vi "LoadScanSettings.vi"(10 "Digitizer Settings In":T1={"Digitizer delay (us) "=0.0, "rf points per line"=2048, "lines per plane"=128, "Samp Rate (Hz)"=100000000.0, "Additional dig delay (us)"=0.0, "Voltage Scale"=0.4, "Pre-Looks"=0, "Offset delay (us)"=0.0, "bits A/D"=8, "Avg Num"=1, "DigTimeOut"=5.0, "Rel Dig Delay"=0.0, "Dig Ch"=0, "LeCroyCluster"={"LeCroy Channels"=[TRUE, FALSE, FALSE, FALSE], "LC read pt offset"=0.0, "Sweep Avg"=FALSE}, "Main Digitizer"=enum."NI Digitizer", "Dig Config"=enum."Single channel", "Digitizer ID Cluster"={"Acqiris/Alazar/SP ID"=[], "NI Instr Handles"=[], "LeCroy VISA"="", "GaGe Handle"={"Handle"=0, "Sample size"=0, "Resolution"=0, "Offset"=0, "Channels"=0, "Boards"=0}, "ATS Ref"="ATS9350", "Acqiris Address"=["PCI::INSTR0"], "ADQRef"=refnum, "adq_cu_ptr"=refnum}, "Trigger Settings"={"Trig Source"=1, "Trig Coupling"=0, "Trig Slope"=0, "Level (mV)"=1500.0}, "Bulk Acq"=FALSE, "Bulk Start Indexes"=[], "Data Ref RF"=refnum, "NI ID/Channel"=[], "Total Dig CH"=5, "Xtra Ann Trig delay (us)"=10.0, "Fix Z Delay?"=FALSE, "One Way Transmission?"=FALSE, "Data Ref Log"=refnum} {"Trigger Settings"."Trig Slope" items=["Positive", "Negative"]; "Trigger Settings"."Level (mV)" format="%.2f"; "Trigger Settings"."Trig Coupling" items=["DC 1 MOhm", "AC 1 MOhm", "DC 50 Ohm", "AC 50 Ohm"]; "Trigger Settings"."Trig Source" items=["Chan 1", "External"]; "Rel Dig Delay" format="%.2f"; "DigTimeOut" format="%.2f"; "Avg Num" min=1; "Offset delay (us)" format="%.2f"; "Additional dig delay (us)" format="%.2f"; "Digitizer delay (us)" format="%.2f"}, 11 "Motion Settings In":T5={"No Motion?"=FALSE, "Motion System"=enum."NI 735x", "Motion Bd ID"=1, "Motion Profile"="SMAC1", "# Axis"=1, "Reverse Z axis?"=TRUE, "SMAC Axis"=0, "scan pair"=enum."y-(x) scan", "RT fps"=6.0, "Steps per mm"=[1000, 1000, 1000, 1000], "Motor Parameters"={"velocity ct/s"=[10000.0, 10000.0, 10000.0, 50000.0], "accel ct/s^2"=[50000.0, 50000.0, 50000.0, 200000.0]}, "One Way Scan"=FALSE, "Reverse One Way Scan"=FALSE, "Global Position (mm)"=[], "Plane"=0, "Distance between\nscan lines (um)"=0.0, "Distance between\nscan planes (um)"=0.0, "number of scan planes"=1, "Total steps in line"=0, "Xtra plane\ndistance  (um)"=100, "Xtra planes "=1, "Add Axis"=FALSE, "overshoot cts"=200, "BKPT Shift"=0, "Scan Start Time (ms)"=0, "ESP VISA"="GPIB::1::INSTR", "3rd Axis"=1, "GL Ref Out"=refnum, "Galil Address"=""} {"3rd Axis" items=["x", "y", "z", "w"]; "Xtra planes" min=1; "Xtra plane\ndistance  (um)" min=0; "Distance between\nscan planes (um)" format="%.2f"; "Distance between\nscan lines (um)" format="%.2f"; "SMAC Axis" items=["None"=0, "Axis 1"=1, "Axis 2"=2, "Axis 3"=3, "Axis 4"=4, "Axis 5"=5, "Axis 6"=6, "Axis 7"=7, "Axis 8"=8, "Vector Space 1"=17, "Vector Space 2"=18, "Vector Space 3"=19, "Vector Space 4"=20]; "Motion Bd ID" min=1 max=32 step=1}) -> (0 "Canceled":bool, 1 "Type of scan out":T13=enum."M scan", 2 "Digitizer Settings out":T1={"Digitizer delay (us) "=0.0, "rf points per line"=2048, "lines per plane"=128, "Samp Rate (Hz)"=100000000.0, "Additional dig delay (us)"=0.0, "Voltage Scale"=0.4, "Pre-Looks"=0, "Offset delay (us)"=0.0, "bits A/D"=8, "Avg Num"=1, "DigTimeOut"=5.0, "Rel Dig Delay"=0.0, "Dig Ch"=0, "LeCroyCluster"={"LeCroy Channels"=[TRUE, FALSE, FALSE, FALSE], "LC read pt offset"=0.0, "Sweep Avg"=FALSE}, "Main Digitizer"=enum."NI Digitizer", "Dig Config"=enum."Single channel", "Digitizer ID Cluster"={"Acqiris/Alazar/SP ID"=[], "NI Instr Handles"=[], "LeCroy VISA"="", "GaGe Handle"={"Handle"=0, "Sample size"=0, "Resolution"=0, "Offset"=0, "Channels"=0, "Boards"=0}, "ATS Ref"="ATS9350", "Acqiris Address"=["PCI::INSTR0"], "ADQRef"=refnum, "adq_cu_ptr"=refnum}, "Trigger Settings"={"Trig Source"=1, "Trig Coupling"=0, "Trig Slope"=0, "Level (mV)"=1500.0}, "Bulk Acq"=FALSE, "Bulk Start Indexes"=[], "Data Ref RF"=refnum, "NI ID/Channel"=[], "Total Dig CH"=5, "Xtra Ann Trig delay (us)"=10.0, "Fix Z Delay?"=FALSE, "One Way Transmission?"=FALSE, "Data Ref Log"=refnum} {"Trigger Settings"."Trig Slope" items=["Positive", "Negative"]; "Trigger Settings"."Level (mV)" format="%.2f"; "Trigger Settings"."Trig Coupling" items=["DC 1 MOhm", "AC 1 MOhm", "DC 50 Ohm", "AC 50 Ohm"]; "Trigger Settings"."Trig Source" items=["Chan 1", "External"]; "Rel Dig Delay" format="%.2f"; "DigTimeOut" format="%.2f"; "Avg Num" min=1; "Offset delay (us)" format="%.2f"; "Additional dig delay (us)" format="%.2f"; "Digitizer delay (us)" format="%.2f"}, 3 "Motion Settings out":T5={"No Motion?"=FALSE, "Motion System"=enum."NI 735x", "Motion Bd ID"=1, "Motion Profile"="SMAC1", "# Axis"=1, "Reverse Z axis?"=TRUE, "SMAC Axis"=0, "scan pair"=enum."y-(x) scan", "RT fps"=6.0, "Steps per mm"=[1000, 1000, 1000, 1000], "Motor Parameters"={"velocity ct/s"=[10000.0, 10000.0, 10000.0, 50000.0], "accel ct/s^2"=[50000.0, 50000.0, 50000.0, 200000.0]}, "One Way Scan"=FALSE, "Reverse One Way Scan"=FALSE, "Global Position (mm)"=[], "Plane"=0, "Distance between\nscan lines (um)"=0.0, "Distance between\nscan planes (um)"=0.0, "number of scan planes"=1, "Total steps in line"=0, "Xtra plane\ndistance  (um)"=100, "Xtra planes "=1, "Add Axis"=FALSE, "overshoot cts"=200, "BKPT Shift"=0, "Scan Start Time (ms)"=0, "ESP VISA"="GPIB::1::INSTR", "3rd Axis"=1, "GL Ref Out"=refnum, "Galil Address"=""} {"3rd Axis" items=["x", "y", "z", "w"]; "Xtra planes" min=1; "Xtra plane\ndistance  (um)" min=0; "Distance between\nscan planes (um)" format="%.2f"; "Distance between\nscan lines (um)" format="%.2f"; "SMAC Axis" items=["None"=0, "Axis 1"=1, "Axis 2"=2, "Axis 3"=3, "Axis 4"=4, "Axis 5"=5, "Axis 6"=6, "Axis 7"=7, "Axis 8"=8, "Vector Space 1"=17, "Vector Space 2"=18, "Vector Space 3"=19, "Vector Space 4"=20]; "Motion Bd ID" min=1 max=32 step=1}, 4 "Panametrics Settings Out":T11={"ENERGY (uJ)"=0, "DAMPING (Ohm)"=0, "HP FILT (KHz) "=0, "LP FILT (MHz)"=0, "MODE"=0, "PRF (KHz)"=1, "GAIN (db)"=0, "COARSE ATTENUATION"=0, "FINE ATTENUATION"=0} {"FINE ATTENUATION" items=["00.0", "00.5", "01.0", "01.5", "02.0", "02.5", "03.0", "03.5", "04.0", "04.5", "05.0", "05.5", "06.0", "06.5", "07.0", "07.5", "08.0", "08.5", "09.0", "09.5", "10.0", "10.5", "11.0", "11.5", "12.0", "12.5", "13.0", "13.5", "14.0", "14.5", "15.0", "15.5"]; "COARSE ATTENUATION" items=["00.0", "10.0", "20.0", "30.0", "40.0", "50.0"]; "GAIN (db)" items=["26.0", "40.0", "54.0"]; "PRF (KHz)" items=["XREMT", "EXBNC", "0.200", "0.500", "1.000", "2.000", "5.000", "10.00", "20.00"]; "MODE" items=["P/ E", "THRU", "RPP", "EXT_PLSR"]; "LP FILT (MHz)" items=["20", "50", "100", "200"]; "HP FILT (KHz)" items=["1", "1000", "3000", "10000"]; "DAMPING (Ohm)" items=["7", "10", "16", "20", "26", "30", "40", "50"]; "ENERGY (uJ)" items=["1", "2", "4", "8", "16", "32"]}, 5 "Daxsonics Settings Out":T10={"Freq (MHz) "=20, "Voltage (V)"=0, "Gain (dB)"=22} {"Freq (MHz)" items=["50"=50, "45"=45, "40"=40, "35"=35, "30"=30, "25"=25, "20"=20, "18"=18, "17"=17, "16"=16, "15"=15, "14"=14, "12"=12, "10"=10, "8"=8, "6"=6, "5"=5, "4"=4]; "Voltage (V)" items=["190"=190, "180"=180, "170"=170, "160"=160, "150"=150, "140"=140, "130"=130, "120"=120, "110"=110, "100"=100, "95"=95, "90"=90, "85"=85, "80"=80, "75"=75, "70"=70, "65"=65, "60"=60, "55"=55, "50"=50, "45"=45, "40"=40, "35"=35, "30"=30, "25"=25, "20"=20, "15"=15, "10"=10, "5"=5, "0"=0]; "Gain (dB)" items=["67"=67, "64"=64, "61"=61, "58"=58, "55"=55, "52"=52, "49"=49, "46"=46, "43"=43, "40"=40, "37"=37, "34"=34, "31"=31, "28"=28, "25"=25, "22"=22]}, 6 "Case Name Modifier Out":string, 8 "Pulser Out":T9)   [LabVIEW 2022 SP3]
uses:
  Controls/ScanType2.ctl
  Motion Controllers/-MotionRoutines/ScanAxis.ctl
  Motion Controllers/NI_controller/-NI_MotionRoutines/MotionParameters.ctl
  Motion Controllers/NI_controller/-NI_MotionRoutines/MotionSys.ctl
  Motion Controllers/-MotionRoutines/3rdAxis.ctl
  Digitizers/-DigitizerRoutines/DigitizerSettings.ctl
  Digitizers/-DigitizerRoutines/Digitizer.ctl
  Digitizers/-DigitizerRoutines/DigConfig.ctl
  Digitizers/-DigitizerRoutines/DigitizerID.ctl
  C:/Windows/System32/ADQAPI_dotNet_helper.dll
  Controls/CompleteScanSettings.ctl
  Pulsers/Panametrics/Pana5900.ctl
  Pulsers/Daxsonics/-DaxSubroutines/Dax_Control_Cluster.ctl
  Pulsers/pulser.ctl
  Motion Controllers/-MotionRoutines/MotionGlobals.vi
  <vilib>/Utility/xml.llb/Read From XML File(string).vi
panel:
  in  "Cancel":bool
  in  "Daxsonics Settings":T10={"Freq (MHz) "=20, "Voltage (V)"=0, "Gain (dB)"=22} {"Freq (MHz)" items=["50"=50, "45"=45, "40"=40, "35"=35, "30"=30, "25"=25, "20"=20, "18"=18, "17"=17, "16"=16, "15"=15, "14"=14, "12"=12, "10"=10, "8"=8, "6"=6, "5"=5, "4"=4]; "Voltage (V)" items=["190"=190, "180"=180, "170"=170, "160"=160, "150"=150, "140"=140, "130"=130, "120"=120, "110"=110, "100"=100, "95"=95, "90"=90, "85"=85, "80"=80, "75"=75, "70"=70, "65"=65, "60"=60, "55"=55, "50"=50, "45"=45, "40"=40, "35"=35, "30"=30, "25"=25, "20"=20, "15"=15, "10"=10, "5"=5, "0"=0]; "Gain (dB)" items=["67"=67, "64"=64, "61"=61, "58"=58, "55"=55, "52"=52, "49"=49, "46"=46, "43"=43, "40"=40, "37"=37, "34"=34, "31"=31, "28"=28, "25"=25, "22"=22]}
  in  "Panametrics Settings":T11={"ENERGY (uJ)"=0, "DAMPING (Ohm)"=0, "HP FILT (KHz) "=0, "LP FILT (MHz)"=0, "MODE"=0, "PRF (KHz)"=1, "GAIN (db)"=0, "COARSE ATTENUATION"=0, "FINE ATTENUATION"=0} {"FINE ATTENUATION" items=["00.0", "00.5", "01.0", "01.5", "02.0", "02.5", "03.0", "03.5", "04.0", "04.5", "05.0", "05.5", "06.0", "06.5", "07.0", "07.5", "08.0", "08.5", "09.0", "09.5", "10.0", "10.5", "11.0", "11.5", "12.0", "12.5", "13.0", "13.5", "14.0", "14.5", "15.0", "15.5"]; "COARSE ATTENUATION" items=["00.0", "10.0", "20.0", "30.0", "40.0", "50.0"]; "GAIN (db)" items=["26.0", "40.0", "54.0"]; "PRF (KHz)" items=["XREMT", "EXBNC", "0.200", "0.500", "1.000", "2.000", "5.000", "10.00", "20.00"]; "MODE" items=["P/ E", "THRU", "RPP", "EXT_PLSR"]; "LP FILT (MHz)" items=["20", "50", "100", "200"]; "HP FILT (KHz)" items=["1", "1000", "3000", "10000"]; "DAMPING (Ohm)" items=["7", "10", "16", "20", "26", "30", "40", "50"]; "ENERGY (uJ)" items=["1", "2", "4", "8", "16", "32"]}
  in  "Pulser":T9
  in  "ScanSettings":T12={"Type of scan"=enum."M scan", "Motion Settings In"={"No Motion?"=FALSE, "Motion System"=enum."NI 735x", "Motion Bd ID"=1, "Motion Profile"="SMAC1", "# Axis"=1, "Reverse Z axis?"=TRUE, "SMAC Axis"=0, "scan pair"=enum."y-(x) scan", "RT fps"=6.0, "Steps per mm"=[1000, 1000, 1000, 1000], "Motor Parameters"={"velocity ct/s"=[10000.0, 10000.0, 10000.0, 50000.0], "accel ct/s^2"=[50000.0, 50000.0, 50000.0, 200000.0]}, "One Way Scan"=FALSE, "Reverse One Way Scan"=FALSE, "Global Position (mm)"=[], "Plane"=0, "Distance between\nscan lines (um)"=0.0, "Distance between\nscan planes (um)"=0.0, "number of scan planes"=1, "Total steps in line"=0, "Xtra plane\ndistance  (um)"=100, "Xtra planes "=1, "Add Axis"=FALSE, "overshoot cts"=200, "BKPT Shift"=0, "Scan Start Time (ms)"=0, "ESP VISA"="GPIB::1::INSTR", "3rd Axis"=1, "GL Ref Out"=refnum, "Galil Address"=""}, "Digitizer Settings"={"Digitizer delay (us) "=0.0, "rf points per line"=2048, "lines per plane"=128, "Samp Rate (Hz)"=100000000.0, "Additional dig delay (us)"=0.0, "Voltage Scale"=0.4, "Pre-Looks"=0, "Offset delay (us)"=0.0, "bits A/D"=8, "Avg Num"=1, "DigTimeOut"=5.0, "Rel Dig Delay"=0.0, "Dig Ch"=0, "LeCroyCluster"={"LeCroy Channels"=[TRUE, FALSE, FALSE, FALSE], "LC read pt offset"=0.0, "Sweep Avg"=FALSE}, "Main Digitizer"=enum."NI Digitizer", "Dig Config"=enum."Single channel", "Digitizer ID Cluster"={"Acqiris/Alazar/SP ID"=[], "NI Instr Handles"=[], "LeCroy VISA"="", "GaGe Handle"={"Handle"=0, "Sample size"=0, "Resolution"=0, "Offset"=0, "Channels"=0, "Boards"=0}, "ATS Ref"="ATS9350", "Acqiris Address"=["PCI::INSTR0"], "ADQRef"=refnum, "adq_cu_ptr"=refnum}, "Trigger Settings"={"Trig Source"=1, "Trig Coupling"=0, "Trig Slope"=0, "Level (mV)"=1500.0}, "Bulk Acq"=FALSE, "Bulk Start Indexes"=[], "Data Ref RF"=refnum, "NI ID/Channel"=[], "Total Dig CH"=1, "Xtra Ann Trig delay (us)"=10.0, "Fix Z Delay?"=FALSE, "One Way Transmission?"=FALSE, "Data Ref Log"=refnum}, "Case Name Modifier"="Case", "Panametrics Settings"={"ENERGY (uJ)"=0, "DAMPING (Ohm)"=0, "HP FILT (KHz) "=0, "LP FILT (MHz)"=0, "MODE"=0, "PRF (KHz)"=1, "GAIN (db)"=0, "COARSE ATTENUATION"=0, "FINE ATTENUATION"=0}, "Daxsonics Settings"={"Freq (MHz) "=20, "Voltage (V)"=0, "Gain (dB)"=22}, "Pulser"=enum."Pan 5900"} {"Daxsonics Settings"."Freq (MHz)" items=["50"=50, "45"=45, "40"=40, "35"=35, "30"=30, "25"=25, "20"=20, "18"=18, "17"=17, "16"=16, "15"=15, "14"=14, "12"=12, "10"=10, "8"=8, "6"=6, "5"=5, "4"=4]; "Daxsonics Settings"."Voltage (V)" items=["190"=190, "180"=180, "170"=170, "160"=160, "150"=150, "140"=140, "130"=130, "120"=120, "110"=110, "100"=100, "95"=95, "90"=90, "85"=85, "80"=80, "75"=75, "70"=70, "65"=65, "60"=60, "55"=55, "50"=50, "45"=45, "40"=40, "35"=35, "30"=30, "25"=25, "20"=20, "15"=15, "10"=10, "5"=5, "0"=0]; "Daxsonics Settings"."Gain (dB)" items=["67"=67, "64"=64, "61"=61, "58"=58, "55"=55, "52"=52, "49"=49, "46"=46, "43"=43, "40"=40, "37"=37, "34"=34, "31"=31, "28"=28, "25"=25, "22"=22]; "Panametrics Settings"."FINE ATTENUATION" items=["00.0", "00.5", "01.0", "01.5", "02.0", "02.5", "03.0", "03.5", "04.0", "04.5", "05.0", "05.5", "06.0", "06.5", "07.0", "07.5", "08.0", "08.5", "09.0", "09.5", "10.0", "10.5", "11.0", "11.5", "12.0", "12.5", "13.0", "13.5", "14.0", "14.5", "15.0", "15.5"]; "Panametrics Settings"."COARSE ATTENUATION" items=["00.0", "10.0", "20.0", "30.0", "40.0", "50.0"]; "Panametrics Settings"."GAIN (db)" items=["26.0", "40.0", "54.0"]; "Panametrics Settings"."PRF (KHz)" items=["XREMT", "EXBNC", "0.200", "0.500", "1.000", "2.000", "5.000", "10.00", "20.00"]; "Panametrics Settings"."MODE" items=["P/ E", "THRU", "RPP", "EXT_PLSR"]; "Panametrics Settings"."LP FILT (MHz)" items=["20", "50", "100", "200"]; "Panametrics Settings"."HP FILT (KHz)" items=["1", "1000", "3000", "10000"]; "Panametrics Settings"."DAMPING (Ohm)" items=["7", "10", "16", "20", "26", "30", "40", "50"]; "Panametrics Settings"."ENERGY (uJ)" items=["1", "2", "4", "8", "16", "32"]; "Digitizer Settings"."Trigger Settings"."Trig Slope" items=["Positive", "Negative"]; "Digitizer Settings"."Trigger Settings"."Level (mV)" format="%.2f"; "Digitizer Settings"."Trigger Settings"."Trig Coupling" items=["DC 1 MOhm", "AC 1 MOhm", "DC 50 Ohm", "AC 50 Ohm"]; "Digitizer Settings"."Trigger Settings"."Trig Source" items=["Chan 1", "External"]; "Digitizer Settings"."Rel Dig Delay" format="%.2f"; "Digitizer Settings"."DigTimeOut" format="%.2f"; "Digitizer Settings"."Avg Num" min=1; "Digitizer Settings"."Offset delay (us)" format="%.2f"; "Digitizer Settings"."Additional dig delay (us)" format="%.2f"; "Digitizer Settings"."Digitizer delay (us)" format="%.2f"; "Motion Settings In"."3rd Axis" items=["x", "y", "z", "w"]; "Motion Settings In"."Xtra planes" min=1; "Motion Settings In"."Xtra plane\ndistance  (um)" min=0; "Motion Settings In"."Distance between\nscan planes (um)" format="%.2f"; "Motion Settings In"."Distance between\nscan lines (um)" format="%.2f"; "Motion Settings In"."SMAC Axis" items=["None"=0, "Axis 1"=1, "Axis 2"=2, "Axis 3"=3, "Axis 4"=4, "Axis 5"=5, "Axis 6"=6, "Axis 7"=7, "Axis 8"=8, "Vector Space 1"=17, "Vector Space 2"=18, "Vector Space 3"=19, "Vector Space 4"=20]; "Motion Settings In"."Motion Bd ID" min=1 max=32 step=1}
  out "Size of one \nRF line (mm)":dbl=128.0 format="%.2f"
  out "Size of all \nplanes (mm)":dbl=128.0 format="%.2f"
  out "Size of one \nplane (mm)":dbl=128.0 format="%.2f"
  in  "Fix Z Delay?":bool
  in  "Voltage Scale":dbl
  in  "Additional dig delay (us)":dbl
  in  "Digitizer delay (us)":dbl
  in  "Samp Rate (MHz)":dbl
  in  "lines per plane":i32
  in  "rf points per line":i32
  in  "number of scan planes":i32
  in  "Distance between\nscan planes (um)":sgl
  in  "Distance between\nscan lines (um)":sgl
  in  "Reverse One Way Scan":bool
  in  "One Way Scan":bool
  in  "scan pair":T7=enum."x-(y) scan"
  in  "save":bool
  in  "Type of scan":T13=enum."M scan"
  in  "Case Name Modifier":string="Case"
  # "Confirm Relevant Settings"
  # "1-D and 2-D B scan settings"
  # "1-D and 2-D B scan settings"
  # "1-D and 2-D B scan settings"
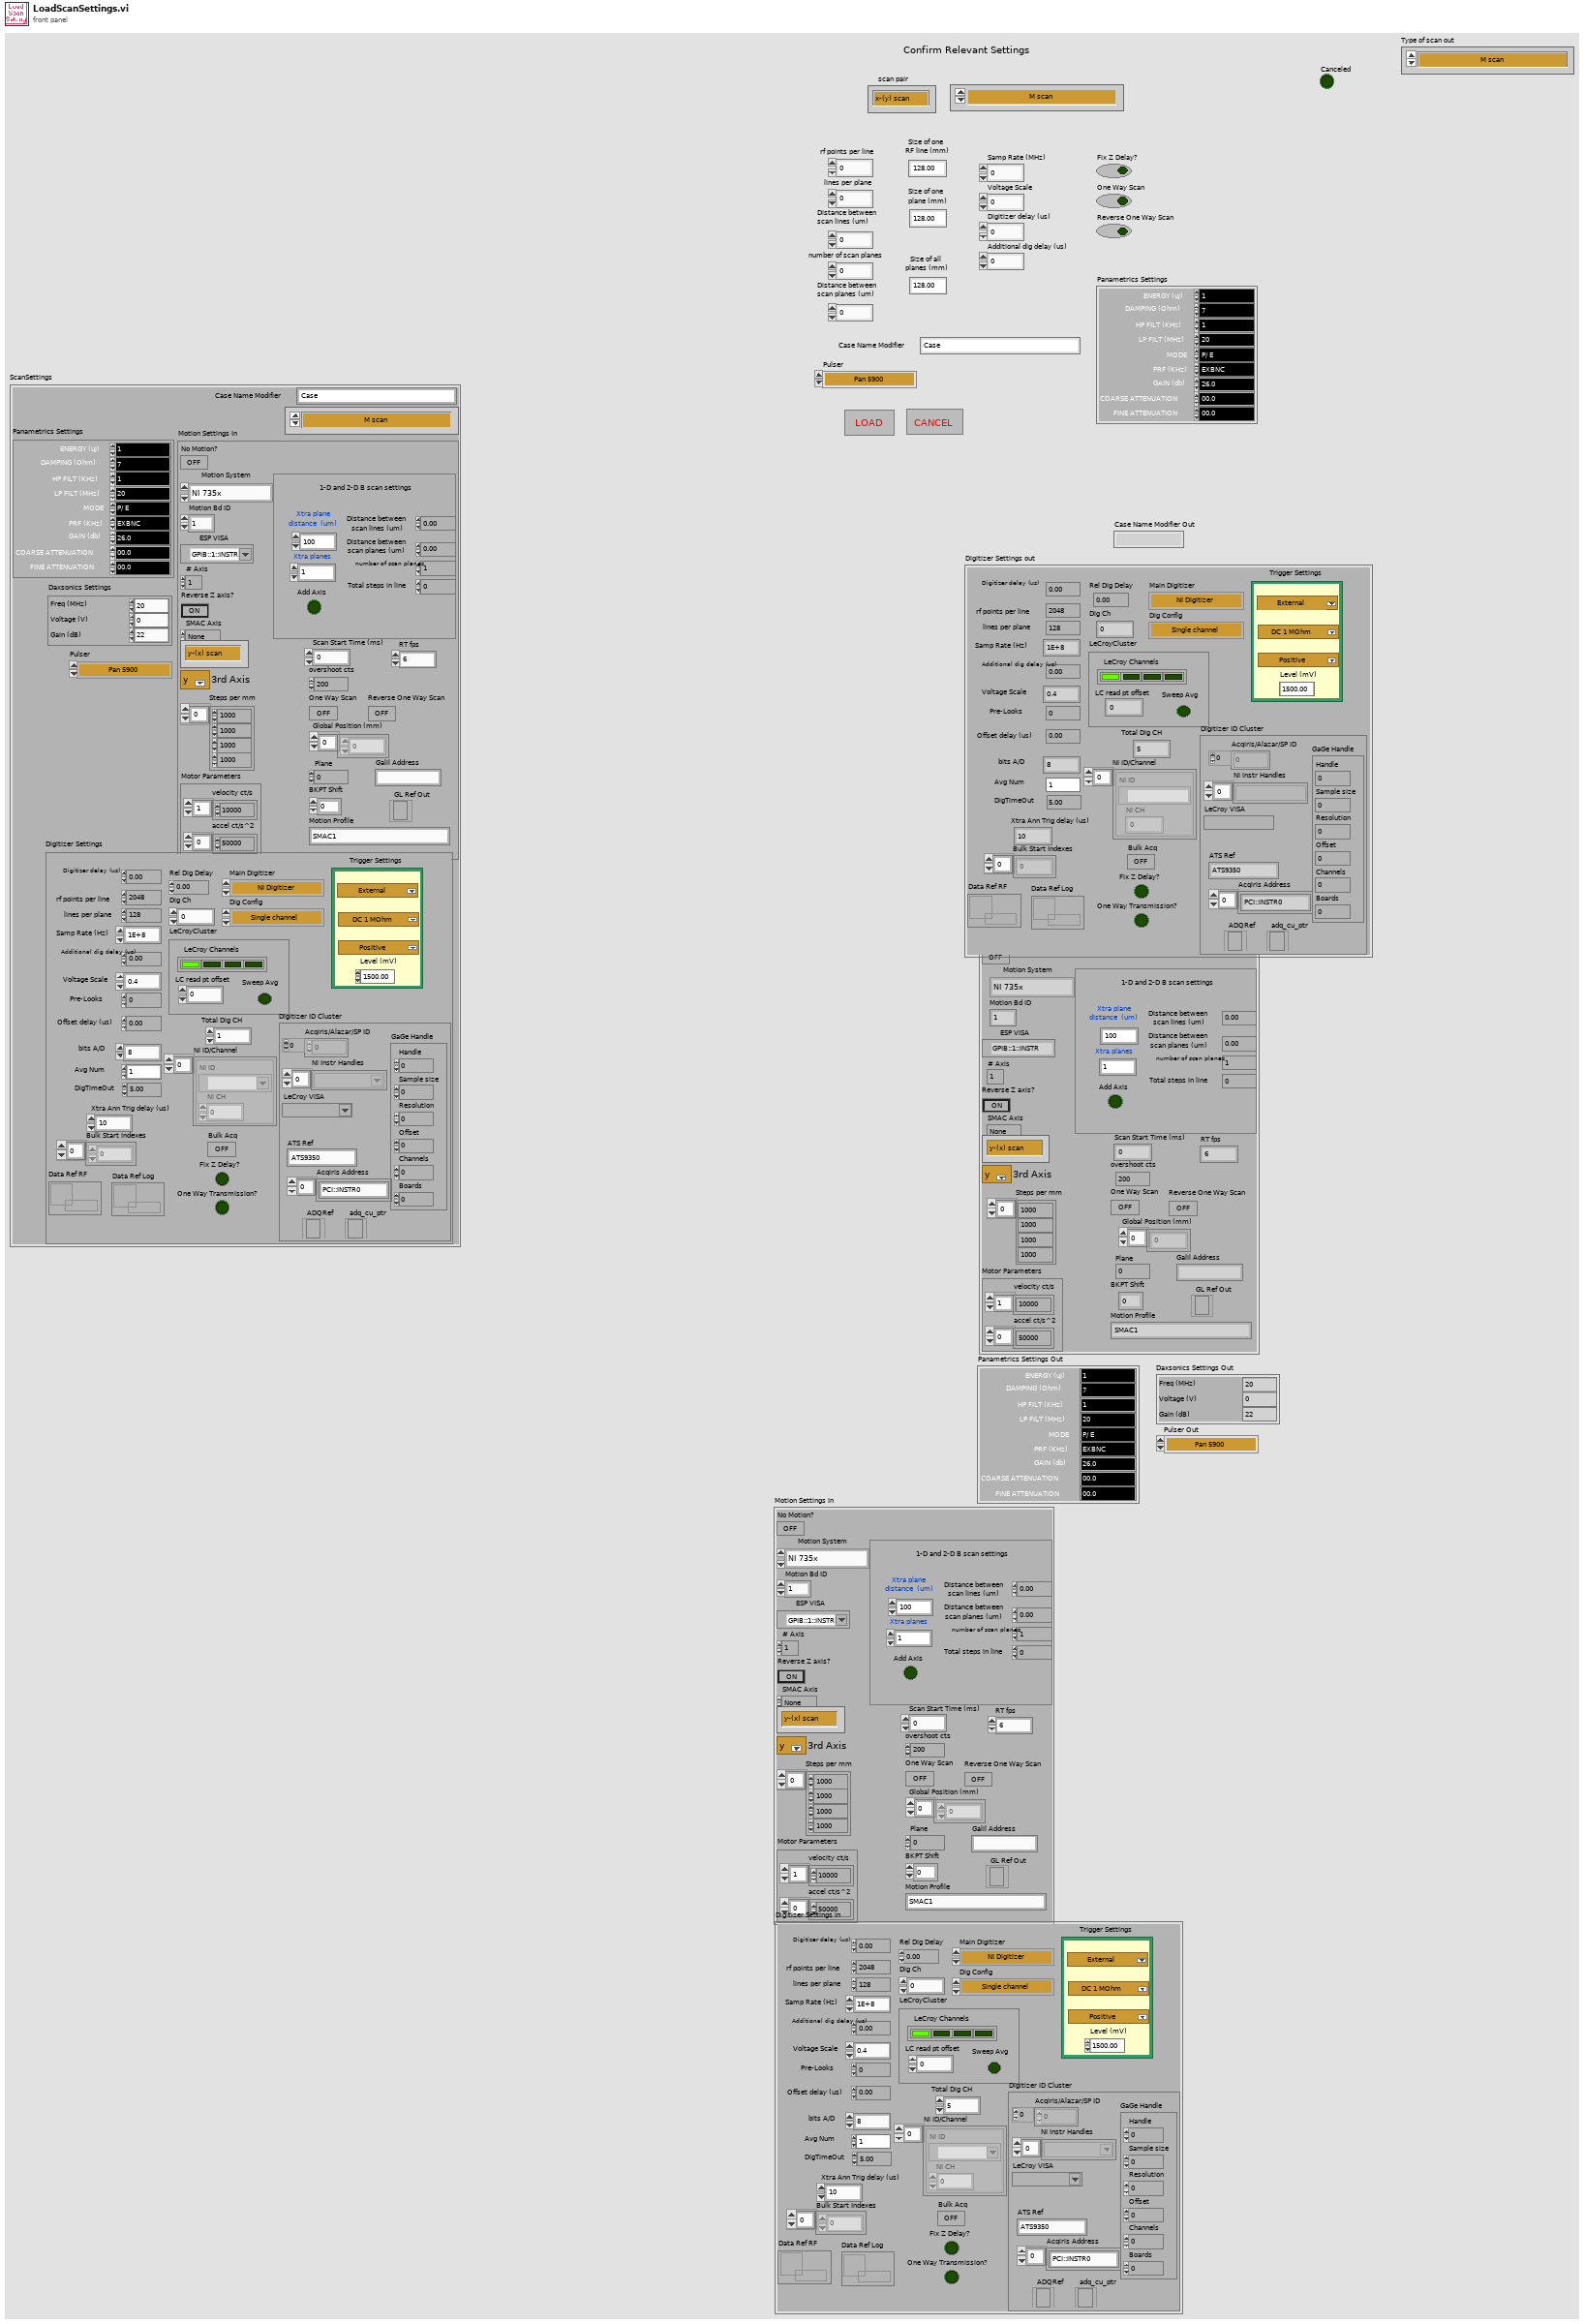
[diagram p1: front panel]
types:
  T1 = typedef "DigitizerSettings.ctl" = cluster{"Digitizer delay (us) ":dbl, "rf points per line":i32, "lines per plane":i32, "Samp Rate (Hz)":dbl, "Additional dig delay (us)":dbl, "Voltage Scale":dbl, "Pre-Looks":i32, "Offset delay (us)":dbl, "bits A/D":i8, "Avg Num":i32, "DigTimeOut":sgl, "Rel Dig Delay":sgl, "Dig Ch":i32, "LeCroyCluster":cluster{"LeCroy Channels":bool[], "LC read pt offset":dbl, "Sweep Avg":bool}, "Main Digitizer":T2, "Dig Config":T3, "Digitizer ID Cluster":T4, "Trigger Settings":cluster{"Trig Source":u16, "Trig Coupling":u16, "Trig Slope":u16, "Level (mV)":dbl}, "Bulk Acq":bool, "Bulk Start Indexes":i32[], "Data Ref RF":refnum<data-value>, "NI ID/Channel":cluster{"NI ID":refnum<k15>, "NI CH":i32}[], "Total Dig CH":i32, "Xtra Ann Trig delay (us)":dbl, "Fix Z Delay?":bool, "One Way Transmission?":bool, "Data Ref Log":refnum<data-value>}
  T2 = typedef "Digitizer.ctl" = enum16{"Acqiris Digitizer", "NI Digitizer", "LeCroy", "GaGe", "AlazarTech", "No Digitizer", "Teledyne"}
  T3 = typedef "DigConfig.ctl" = enum16{"Single channel", "2 Chans w/ 2 Acqiris", "2 Chans w/ 1 Acqiris", "5-CH Pulser New", "5-CH pulser w/ ann array", "5-pass style ann array", "Empty"}
  T4 = typedef "DigitizerID.ctl" = cluster{"Acqiris/Alazar/SP ID":u32[], "NI Instr Handles":refnum<k15>[], "LeCroy VISA":refnum<visa-resource-name>, "GaGe Handle":cluster{"Handle":u32, "Sample size":u32, "Resolution":i32, "Offset":i32, "Channels":u32, "Boards":u32}, "ATS Ref":string, "Acqiris Address":string[], "ADQRef":refnum<k24>, "adq_cu_ptr":refnum<k24>}
  T5 = typedef "MotionParameters.ctl" = cluster{"No Motion?":bool, "Motion System":T6, "Motion Bd ID":u8, "Motion Profile":string, "# Axis":i8, "Reverse Z axis?":bool, "SMAC Axis":u16, "scan pair":T7, "RT fps":sgl, "Steps per mm":i32[], "Motor Parameters":cluster{"velocity ct/s":dbl[], "accel ct/s^2":dbl[]}, "One Way Scan":bool, "Reverse One Way Scan":bool, "Global Position (mm)":dbl[], "Plane":i32, "Distance between\nscan lines (um)":sgl, "Distance between\nscan planes (um)":sgl, "number of scan planes":i32, "Total steps in line":i32, "Xtra plane\ndistance  (um)":i32, "Xtra planes ":i32, "Add Axis":bool, "overshoot cts":i32, "BKPT Shift":i32, "Scan Start Time (ms)":u32, "ESP VISA":refnum<visa-resource-name>, "3rd Axis":T8, "GL Ref Out":refnum<k7>, "Galil Address":string}
  T6 = typedef "MotionSys.ctl" = enum16{"MM3000", "NI 735x", "Newport ESP", "No Motion Card", "Galil"}
  T7 = typedef "ScanAxis.ctl" = enum16{"y-(x) scan", "x-(y) scan", "z-(x) scan", "z-(y) scan", "y-(z) scan", "x-(z) scan", "w-(x) scan", "w-(y) scan", "w-(z) scan", "x-(w) scan", "y-(w) scan", "z-(w) scan"}
  T8 = typedef "3rdAxis.ctl" = u16
  T9 = typedef "pulser.ctl" = enum16{"Pan 5900", "Daxsonics", "Agilent 33xxx", "UTEX", "JSR", "WMC Mono-Cycle", "No Pulser", "NYU AVTECH", "Tabor W1281A", "Pan 5800", "Unlisted", "Tabor WX2182B"}
  T10 = typedef "Dax_Control_Cluster.ctl" = cluster{"Freq (MHz) ":u16, "Voltage (V)":u16, "Gain (dB)":u16}
  T11 = typedef "Pana5900.ctl" = cluster{"ENERGY (uJ)":u16, "DAMPING (Ohm)":u16, "HP FILT (KHz) ":u16, "LP FILT (MHz)":u16, "MODE":u16, "PRF (KHz)":u16, "GAIN (db)":u16, "COARSE ATTENUATION":u16, "FINE ATTENUATION":u16}
  T12 = typedef "CompleteScanSettings.ctl" = cluster{"Type of scan":T13, "Motion Settings In":T5, "Digitizer Settings":T1, "Case Name Modifier":string, "Panametrics Settings":T11, "Daxsonics Settings":T10, "Pulser":T9}
  T13 = typedef "ScanType2.ctl" = enum16{"Therapy With Scan", "M scan", "M Scan With Therapy Burst", "1-D B Scan", "1-D B Scan With Therapy Burst", "2-D B Scan", "2-D B Scan With Therapy Burst", "Rotational Scan", "1-D B-Scan PRF", "2-D B-Scan PRF", "Real-Time Scan", "Contrast Agents", "1-D w/ Real-Time Set Up", "Dual Transducer", "Acoustic Microscopy", "Hydrophone Scanning"}
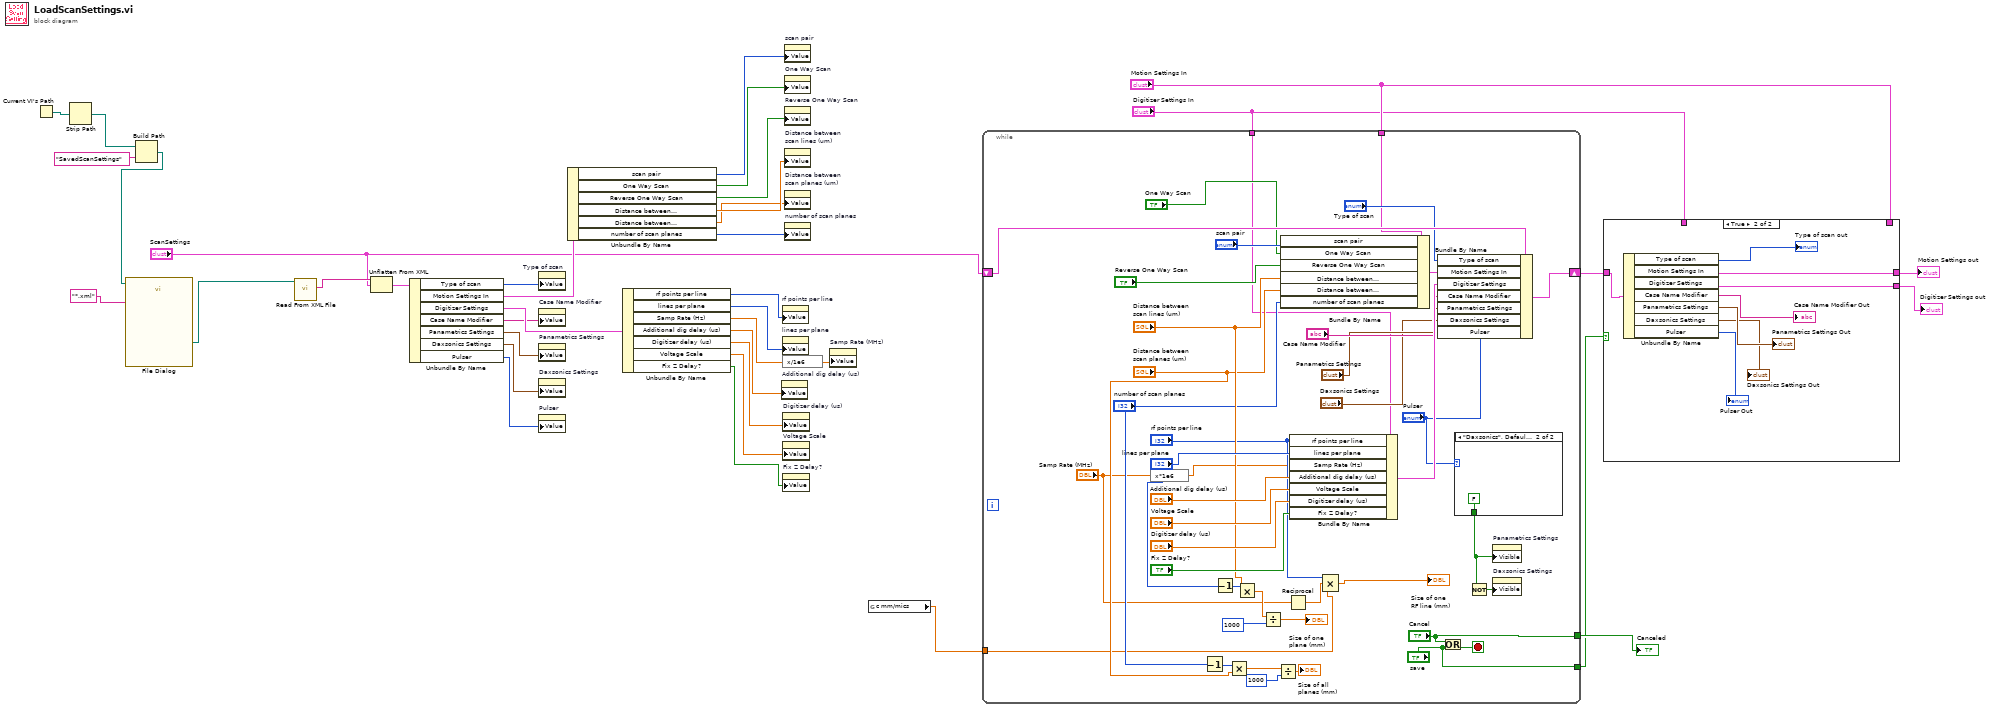
[diagram p0: block diagram]
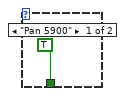
[diagram p3: hidden frame]
diagram:
  n1 = Current VI's Path() -> (path=w9:path)
  n2 = Strip Path(path=w9) -> (stripped path=w8:path)  [unwired: 1 out]
  n3 = Build Path(base path=w8, name or relative path="SavedScanSettings") -> (appended path=w7:path)
  n4 = call "File Dialog"("start path"=w7, "pattern (all files)"="*.xml") -> ("selected path"=w6:path)  [unwired: 10 in, 3 out]
  n5 = call-poly <vilib>:"Read From XML File.vi"("XML File Path"=w6) -> ("XML Elements"=w20:string)  [unwired: 8 in, 2 out]
  n6 = Unflatten From XML(xml string=w20, type="ScanSettings") -> (value=w19:T12)  [unwired: 1 in, 1 out]
  n7 = Unbundle By Name(w19) -> ("Type of scan"=w16:T13, "Motion Settings In"=w18:T5, "Digitizer Settings"=w17:T1, "Case Name Modifier"=w15:string, "Panametrics Settings"=w12:T11, "Daxsonics Settings"=w11:T10, "Pulser"=w13:T9)
  n8 = property on="Type of scan" class="Enum (strict)"("Value"=w16) -> ()  [unwired: 2 in, 2 out]
  n9 = property on="Case Name Modifier" class="Str"("Value"=w15) -> ()  [unwired: 2 in, 2 out]
  n10 = property on="Panametrics Settings" class="Clust (strict)"("Value"=w12) -> ()  [unwired: 2 in, 2 out]
  n11 = property on="Daxsonics Settings" class="Clust (strict)"("Value"=w11) -> ()  [unwired: 2 in, 2 out]
  n12 = property on="Pulser" class="Enum (strict)"("Value"=w13) -> ()  [unwired: 2 in, 2 out]
  n13 = Unbundle By Name(w18) -> ("scan pair"=w38:T7, "One Way Scan"=w37:bool, "Reverse One Way Scan"=w36:bool, "Distance between\nscan lines (um)"=w35:sgl, "Distance between\nscan planes (um)"=w34:sgl, "number of scan planes"=w33:i32)
  n14 = Unbundle By Name(w17) -> ("rf points per line"=w32:i32, "lines per plane"=w31:i32, "Samp Rate (Hz)"=w30:dbl, "Additional dig delay (us)"=w28:dbl, "Digitizer delay (us)"=w27:dbl, "Voltage Scale"=w26:dbl, "Fix Z Delay?"=w25:bool)
  n15 = property on="Additional dig delay (us)" class="DigNum (strict)"("Value"=w28) -> ()  [unwired: 2 in, 2 out]
  n16 = property on="rf points per line" class="DigNum (strict)"("Value"=w32) -> ()  [unwired: 2 in, 2 out]
  n17 = property on="lines per plane" class="DigNum (strict)"("Value"=w31) -> ()  [unwired: 2 in, 2 out]
  n18 = expression code="x/1e6"(w30) -> (w29:dbl)
  n19 = property on="Digitizer delay (us)" class="DigNum (strict)"("Value"=w27) -> ()  [unwired: 2 in, 2 out]
  n20 = property on="Voltage Scale" class="DigNum (strict)"("Value"=w26) -> ()  [unwired: 2 in, 2 out]
  n21 = property on="Fix Z Delay?" class="Bool (strict)"("Value"=w25) -> ()  [unwired: 2 in, 2 out]
  n22 = property on="scan pair" class="Enum (strict)"("Value"=w38) -> ()  [unwired: 2 in, 2 out]
  n23 = property on="One Way Scan" class="Bool (strict)"("Value"=w37) -> ()  [unwired: 2 in, 2 out]
  n24 = property on="Reverse One Way Scan" class="Bool (strict)"("Value"=w36) -> ()  [unwired: 2 in, 2 out]
  n25 = property on="Distance between\nscan lines (um)" class="DigNum (strict)"("Value"=w35) -> ()  [unwired: 2 in, 2 out]
  n26 = property on="Distance between\nscan planes (um)" class="DigNum (strict)"("Value"=w34) -> ()  [unwired: 2 in, 2 out]
  n27 = property on="number of scan planes" class="DigNum (strict)"("Value"=w33) -> ()  [unwired: 2 in, 2 out]
  n28 = property on="Samp Rate (MHz)" class="DigNum (strict)"("Value"=w29) -> ()  [unwired: 2 in, 2 out]
  n29 = global read "MotionGlobals.vi" "c mm/mics"() -> (w21:sgl)
  n30 = while {
    shift-right: [w78] -> w24
    shift-left: "ScanSettings" -> [w79]
    tunnel: w21 -> [w51]
    tunnel: ["save"] -> w3
    tunnel: ["Cancel"] -> w4
    tunnel: "Motion Settings In" -> [w40]
    tunnel: "Digitizer Settings In" -> [w39]
    stop <- w43 stop-if-true
    n31 = expression code="x*1e6"("Samp Rate (MHz)") -> (w53:dbl)
    n32 = Decrement(x="number of scan planes") -> (x-1=w61:i32)
    n33 = Decrement(x="lines per plane") -> (x-1=w66:i32)
    n34 = Multiply(x=w61, y="Distance between\nscan planes (um)") -> (x*y=w60:sgl)
    n35 = Multiply(x=w66, y="Distance between\nscan lines (um)") -> (x*y=w63:sgl)
    n36 = Divide(x=w63, y=1000 ("x")) -> (x/y=→"Size of one \nplane (mm)":sgl)
    n37 = Divide(x=w60, y=1000 ("x")) -> (x/y=→"Size of all \nplanes (mm)":sgl)
    n38 = Bundle By Name(cluster=w40, "scan pair"="scan pair", "One Way Scan"="One Way Scan", "Reverse One Way Scan"="Reverse One Way Scan", "Distance between\nscan lines (um)"="Distance between\nscan lines (um)", "Distance between\nscan planes (um)"="Distance between\nscan planes (um)", "number of scan planes"="number of scan planes") -> (w77:T5)
    n39 = Reciprocal(x="Samp Rate (MHz)") -> (1/x=w54:dbl)
    n40 = Bundle By Name(cluster=w39, "rf points per line"="rf points per line", "lines per plane"="lines per plane", "Samp Rate (Hz)"=w53, "Additional dig delay (us)"="Additional dig delay (us)", "Voltage Scale"="Voltage Scale", "Digitizer delay (us)"="Digitizer delay (us)", "Fix Z Delay?"="Fix Z Delay?") -> (w73:T1)
    n41 = Compound Arithmetic op=MULTIPLY("rf points per line", w54, w51) -> (→"Size of one \nRF line (mm)":dbl)
    n42 = Bundle By Name(cluster=w79, "Type of scan"="Type of scan", "Motion Settings In"=w77, "Digitizer Settings"=w73, "Case Name Modifier"="Case Name Modifier", "Panametrics Settings"="Panametrics Settings", "Daxsonics Settings"="Daxsonics Settings", "Pulser"="Pulser") -> (w78:T12)
    n43 = Or(x="Cancel", y="save") -> (x .or. y?=w43:bool)
    n44 = case shown="\"Daxsonics\", Default" "Pulser" {
      tunnel: [TRUE FALSE] -> w47
      frame "Pan 5900" {
      }
      frame "Daxsonics", Default {
      }
    }
    n45 = Not(x=w47) -> (.not. x?=w46:bool)
    n46 = property on="Panametrics Settings" class="Clust (strict)"("Visible"=w47) -> ()  [unwired: 2 in, 2 out]
    n47 = property on="Daxsonics Settings" class="Clust (strict)"("Visible"=w46) -> ()  [unwired: 2 in, 2 out]
  }
  "Canceled" <- w4
  n48 = case shown="True" w3 {
    tunnel: w24 -> [_ w91]
    tunnel: [w83 w89] -> w23
    tunnel: [w82 w88] -> w22
    tunnel: "Motion Settings In" -> [w83 _]
    tunnel: "Digitizer Settings In" -> [w82 _]
    frame False {
    }
    frame True {
      n49 = Unbundle By Name(w91) -> ("Type of scan"=→"Type of scan out":T13, "Motion Settings In"=w89:T5, "Digitizer Settings"=w88:T1, "Case Name Modifier"=→"Case Name Modifier Out":string, "Panametrics Settings"=→"Panametrics Settings Out":T11, "Daxsonics Settings"=→"Daxsonics Settings Out":T10, "Pulser"=→"Pulser Out":T9)
    }
  }
  "Motion Settings out" <- w23
  "Digitizer Settings out" <- w22
